vi "CC Observation Generate Exposure Step.vi"(8 "error in (no error)":errorcluster, 10 "Images":i32, 11 "Integration Time":dbl) -> (0 "error out":errorcluster, 2 "Exp Name":string="Auto", 3 "Exp Step":T1={"Action"=enum."Acquire Images", "Data"=variant})   [LabVIEW 2024]
uses:
  typedefs/CC Script Step.ctl
  typedefs/CC enum Script Action.ctl
  typedefs/CC cluster Exposure.ctl
  Detector/Detector Class/Detector enum Detector Integration Mode.ctl
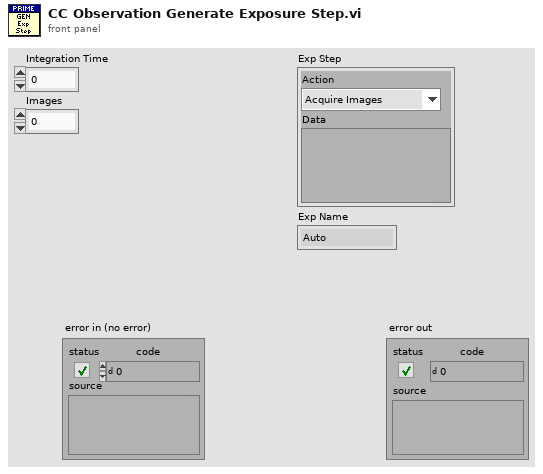
[diagram p1: front panel]
types:
  T1 = typedef "CC Script Step.ctl" = cluster{"Action":T2, "Data":variant}
  T2 = typedef "CC enum Script Action.ctl" = enum16{"Noop", "Define Object", "Define Exposure", "Define Dithering", "Acquire Images", "Set Filter Wheel", "Telescope Home", "Telescope Move", "Telescope RA DEC", "Focus Move Relative", "Focus Move Absolute", "Focus Set Home", "Macro", "Pause", "Ask User", "Define Random Dither", "CmdLine", "Outlet"}
  T3 = typedef "Detector enum Detector Integration Mode.ctl" = enum16{"Ramp", "CDS", "FOWLER2", "FOWLER4", "FOWLER8", "FOWLER16", "Raw"}
  T4 = typedef "CC cluster Exposure.ctl" = cluster{"Mode":T3, "Integration Time":dbl, "Name":string, "Images":i32}
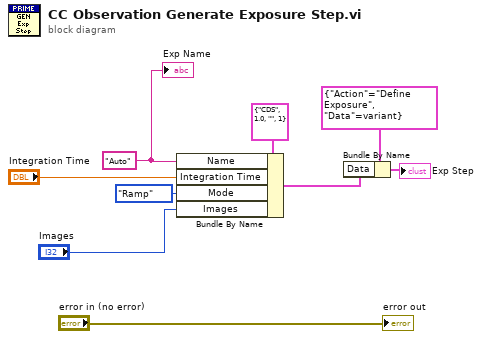
[diagram p0: block diagram]
diagram:
  w5 = "Auto" ("Name")
  n1 = Bundle By Name(cluster=T4 {"Mode"=enum."CDS", "Integration Time"=1.0, "Name"="", "Images"=1} ("value"), "Name"=w5, "Integration Time"="Integration Time", "Mode"=Detector_enum_Detector_Integration_Mode."Ramp", "Images"="Images") -> (w7:T4)
  n2 = Bundle By Name(cluster=T1 {"Action"=enum."Define Exposure", "Data"=variant} ("Cluster"), "Data"=w7) -> (→"Exp Step":T1)
  "error out" <- "error in (no error)"
  "Exp Name" <- w5
